vi "Post-Install Custom Action.vi"(10 "Variant":variant) -> (0 "error out":errorcluster)   [LabVIEW 2013]
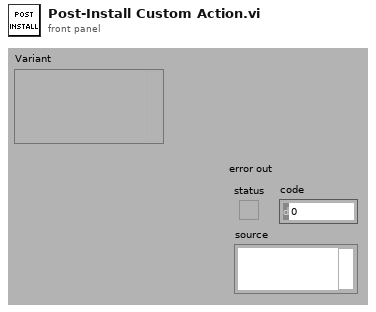
[diagram p1: front panel]
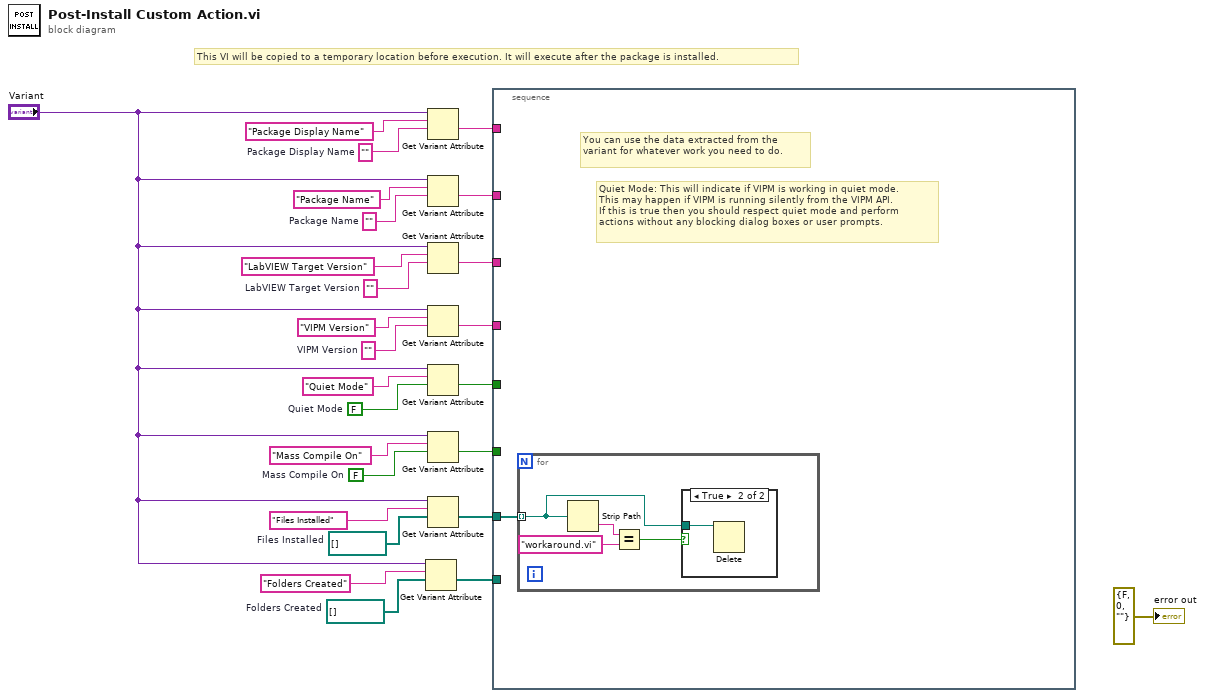
[diagram p0: block diagram]
diagram:
  w1 = path[] []  # Folders Created
  w2 = path[] []  # Files Installed
  w8 = FALSE  # Mass Compile On
  w9 = ""  # Package Display Name
  w16 = FALSE  # Quiet Mode
  w19 = ""  # VIPM Version
  w21 = ""  # LabVIEW Target Version
  w23 = ""  # Package Name
  # "This VI will be copied to a temporary location before execution. It will execute after the package is installed."
  n1 = Get Variant Attribute(Variant="Variant", name="Folders Created", default value (empty Variant)=w1) -> (value=w6:path[])  [unwired: 1 in, 3 out]
  n2 = Get Variant Attribute(Variant="Variant", name="Package Display Name", default value (empty Variant)=w9) -> (value=w15:string)  [unwired: 1 in, 3 out]
  n3 = Get Variant Attribute(Variant="Variant", name="Package Name", default value (empty Variant)=w23) -> (value=w14:string)  [unwired: 1 in, 3 out]
  n4 = Get Variant Attribute(Variant="Variant", name="LabVIEW Target Version", default value (empty Variant)=w21) -> (value=w13:string)  [unwired: 1 in, 3 out]
  n5 = Get Variant Attribute(Variant="Variant", name="VIPM Version", default value (empty Variant)=w19) -> (value=w12:string)  [unwired: 1 in, 3 out]
  n6 = Get Variant Attribute(Variant="Variant", name="Quiet Mode", default value (empty Variant)=w16) -> (value=w11:bool)  [unwired: 1 in, 3 out]
  n7 = Get Variant Attribute(Variant="Variant", name="Mass Compile On", default value (empty Variant)=w8) -> (value=w10:bool)  [unwired: 1 in, 3 out]
  n8 = Get Variant Attribute(Variant="Variant", name="Files Installed", default value (empty Variant)=w2) -> (value=w5:path[])  [unwired: 1 in, 3 out]
  n9 = stacked-sequence {
    tunnel: w15 -> [_]
    tunnel: w14 -> [_]
    tunnel: w13 -> [_]
    tunnel: w12 -> [_]
    tunnel: w11 -> [_]
    tunnel: w10 -> [_]
    tunnel: w5 -> [w27]
    tunnel: w6 -> [_]
    frame #0 {
      # "Quiet Mode: This will indicate if VIPM is working in quiet mode.\nThis may happen if VIPM is running silently from the VIPM API.\nIf this is true then you should respect quiet mode and perform\nactions without any blocking dialog boxes or user prompts."
      # "You can use the data extracted from the variant for whatever work you need to do."
      n10 = for {
        tunnel: w27 -> [w29] mode=indexing
        n11 = Strip Path(path=w29) -> (name=w31:string)  [unwired: 1 out]
        n12 = Equal?(x=w31, y="workaround.vi") -> (x = y?=w28:bool)
        n13 = case shown="True" w28 {
          tunnel: w29 -> [_ w32]
          frame False {
          }
          frame True {
            n14 = Delete(path (use dialog)=w32) -> ()  [unwired: 4 in, 3 out]
          }
        }
      }
    }
  }
  "error out" <- errorcluster {"status"=FALSE, "code"=0, "source"=""} ("error out")
